vi "Get QuickMode From Test Step.vi"(8 "error in (no error)":errorcluster, 9 "Test Configuration (\"\")":string, 11 "Test_ID (\"\")":string) -> (0 "error out":errorcluster, 3 "QuickMode":i8)   [LabVIEW 2011]
uses:
  Test Function.ctl
  Test Return Parameter.ctl
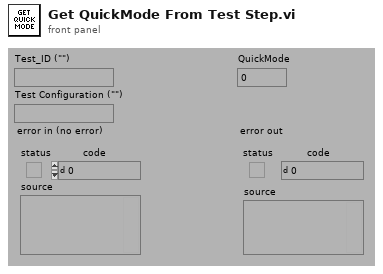
[diagram p1: front panel]
types:
  T1 = typedef "Test Function.ctl" = enum16{"Test Config", "Test Storage", "Test Pre-Process", "Unflatten Test Parameters", "Flatten Test Parameters"}
  T2 = typedef "Test Return Parameter.ctl" = enum16{"Test Parameters", "Required Instruments", "Datasheets", "QuickMode"}
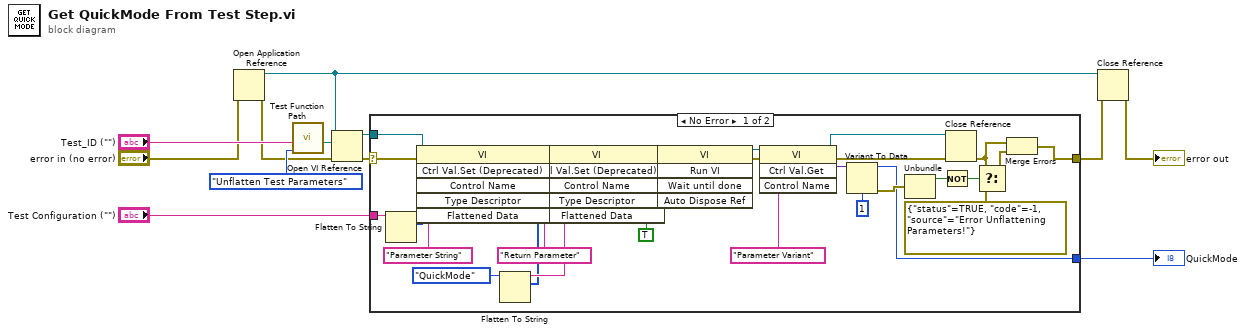
[diagram p0: block diagram]
diagram:
  n1 = Open Application Reference(8:"error in (no error)") -> (0:w1:errorcluster, 3:w3:refnum<vi>)  [unwired: 3 in]
  n2 = call "Test Function Path.vi"("Object Type (Test Config)"=Test_Function."Unflatten Test Parameters", "Object Name (\"\")"="Test_ID (\"\")") -> ("Object Path"=w8:path)  [unwired: 1 in, 8 out]
  n3 = Open VI Reference(application reference (local)=w3, vi path=w8, error in (no error)=w1) -> (vi reference=w10:refnum<vi>, error out=w11:errorcluster)  [unwired: 1 in, 2 out]
  n4 = case shown="No Error" w11 {
    selector: w11 -> [w42 w43]
    tunnel: w10 -> [w41 _]
    tunnel: "Test Configuration (\"\")" -> [w30 _]
    tunnel: [w34 w43] -> w4
    tunnel: [w23 _] -> w6
    frame No Error {
      n5 = Flatten To String(anything=w30) -> (data string=w29:string, type string=w16:i16[])  [unwired: 1 in, 3 out]
      n6 = invoke class="VI" method="Ctrl Val.Set (Deprecated)"(reference=w41, error in=w42, "Control Name"="Parameter String", "Type Descriptor"=w16, "Flattened Data"=w29) -> (reference out=w21:refnum<vi>, error out=w22:errorcluster)  [unwired: 1 in, 4 out]
      n7 = Flatten To String(anything=Test_Return_Parameter."QuickMode" ("Return Parameter")) -> (data string=w18:string, type string=w15:i16[])  [unwired: 1 in, 3 out]
      n8 = invoke class="VI" method="Ctrl Val.Set (Deprecated)"(reference=w21, error in=w22, "Control Name"="Return Parameter", "Type Descriptor"=w15, "Flattened Data"=w18) -> (reference out=w20:refnum<vi>, error out=w19:errorcluster)  [unwired: 1 in, 4 out]
      n9 = invoke class="VI" method="Run VI"(reference=w20, error in=w19, "Wait until done"=TRUE) -> (reference out=w37:refnum<vi>, error out=w38:errorcluster)  [unwired: 2 in, 3 out]
      n10 = invoke class="VI" method="Ctrl Val.Get"(reference=w37, error in=w38, "Control Name"="Parameter Variant") -> (reference out=w35:refnum<vi>, error out=w36:errorcluster, "Get Control Value Variant"=w25:variant)  [unwired: 1 in, 1 out]
      n11 = Variant To Data(type=i8 1 ("QuickMode"), Variant=w25) -> (data=w23:i8, error out=w24:errorcluster)  [unwired: 1 in]
      n12 = Unbundle(w24) -> ("status"=w28:bool)  [unwired: 2 out]
      n13 = Not(x=w28) -> (.not. x?=w27:bool)
      n14 = Close Reference(reference=w35, error in (no error)=w36) -> (error out=w31:errorcluster)
      n15 = Select(t=w31, s=w27, f=errorcluster {"status"=TRUE, "code"=-1, "source"="Error Unflattening Parameters!"}) -> (s? t:f=w32:errorcluster)
      n16 = Merge Errors(w31, w32) -> (w34:errorcluster)
    }
    frame Error {
    }
  }
  "QuickMode" <- w6
  n17 = Close Reference(reference=w3, error in (no error)=w4) -> (error out=→"error out":errorcluster)
